vi "Get Targets_Do.vi"(8 "error in (no error)":errorcluster, 11 "Dependency Source in":refnum<class "Dependency Source.lvclass">) -> (0 "error out":errorcluster, 1 "Success?":bool, 2 "External Target Map":map{string, string}(c390), 3 "Internal Target Map":map{string, string}(c390), 4 "Unhandled Targets":string[](array[string]))   [LabVIEW 2019, in "Project.Dependencies Finder.lvlib" / "Dependency Source.lvclass"]
doc: "Get internal and external targets for the dependency source.\n\nThe default implementation does nothing."
uses:
  Dependency Source.lvclass
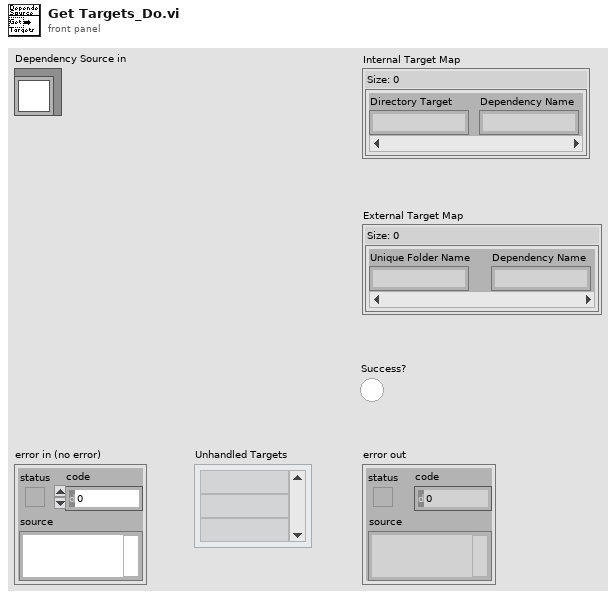
[diagram p1: front panel]
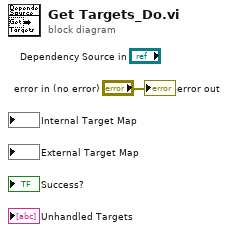
[diagram p0: block diagram]
diagram:
  "error out" <- "error in (no error)"
